vi "Get Vi Memory Name.vi"(8 "error in (no error)":errorcluster, 11 "VI in":refnum<vi>) -> (0 "error out":errorcluster, 2 "Memory Name":string, 3 "VI out":refnum<vi>)   [LabVIEW 2017]
doc: "Returns the in-memory name of the VI wired to VI in, which is how two VIs that share a file name can be told apart."
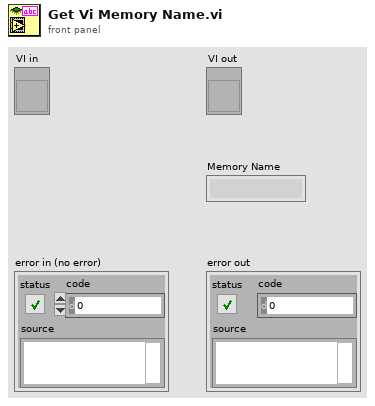
[diagram p1: front panel]
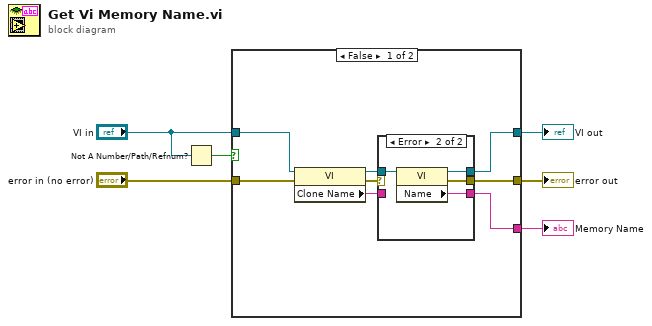
[diagram p0: block diagram]
diagram:
  n1 = Not A Number/Path/Refnum?(number/path/refnum="VI in") -> (NaN/Path/Refnum?=w1:bool)
  n2 = case shown="False" w1 {
    tunnel: [w14 w23] -> w6
    tunnel: [w13 w22] -> w5
    tunnel: "error in (no error)" -> [w12 w22]
    tunnel: [w8 _] -> w3
    tunnel: "VI in" -> [w7 w23]
    frame False {
      n3 = property class="VI"(reference=w7, error in=w12) -> (reference out=w9:refnum<vi>, error out=w10:errorcluster, "Clone Name"=w11:string)
      n4 = case shown="Error" w10 {
        selector: w10 -> [w15 _]
        tunnel: w9 -> [w16 w21]
        tunnel: w11 -> [w17 _]
        tunnel: [w17 w20] -> w8
        tunnel: [w16 w19] -> w14
        tunnel: [w15 w18] -> w13
        frame No Error {
        }
        frame Error {
          n5 = property class="VI"(reference=w21) -> (reference out=w19:refnum<vi>, error out=w18:errorcluster, "Name"=w20:string)  [unwired: 1 in]
        }
      }
    }
    frame True {
    }
  }
  "VI out" <- w6
  "error out" <- w5
  "Memory Name" <- w3
